vi "ToyForStableDisplayOnGrabberAndSavingData2.vi"() -> ()   [LabVIEW 2010]
panel:
  out "Array of 10":u32[](array[numeric])
  in  "Scanning":bool
  out "appended array":u32[](array[numeric])
  out "Remaining array":u32[](array[numeric])
  in  "stop":bool
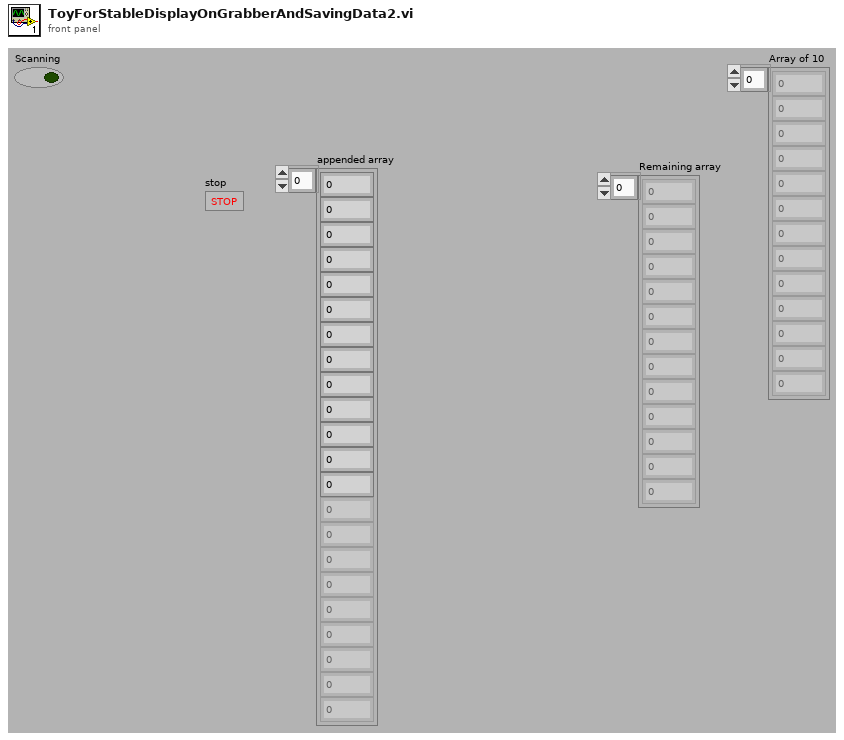
[diagram p1: front panel]
types:
  T1 = enum16{"open", "replace", "create", "open or create", "replace or create", "replace or create with confirmation"}
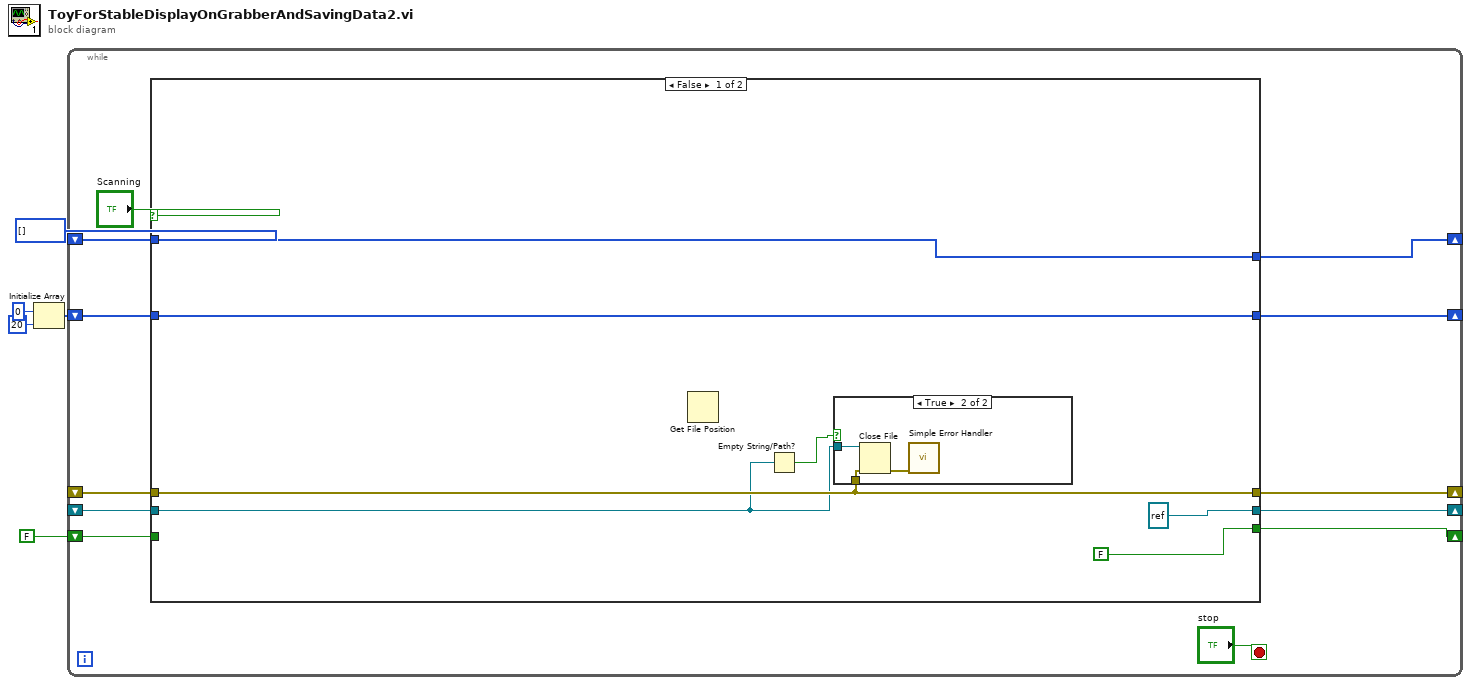
[diagram p0: block diagram]
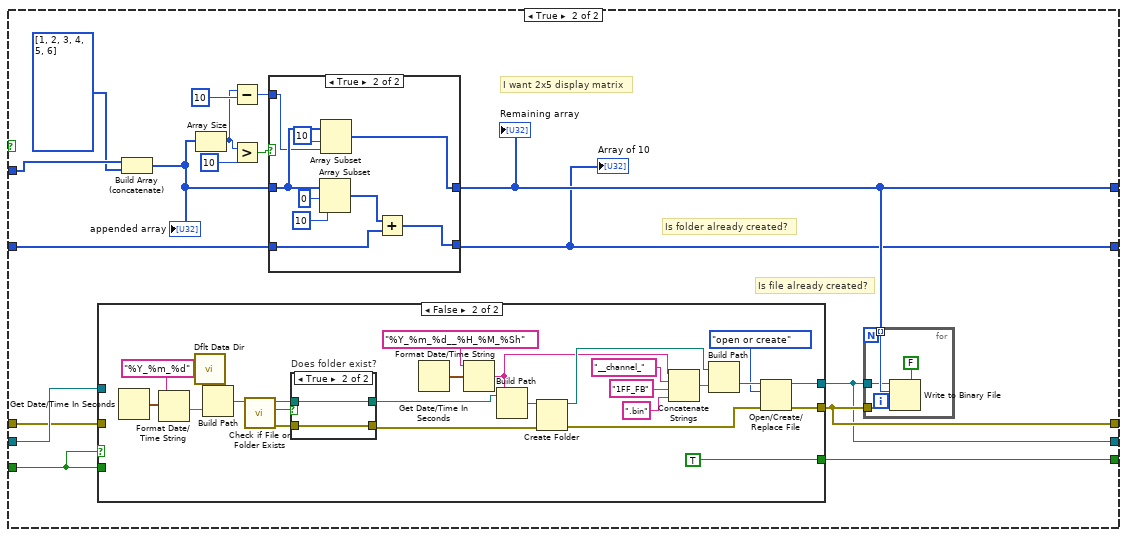
[diagram p3: hidden frame]
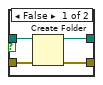
[diagram p5: hidden frame]
diagram:
  n1 = Initialize Array(u32 0 ("element"), 20 ("dimension size")) -> (w2:u32[])
  n2 = while {
    shift-right: [w15] -> _
    shift-left: u32[] [] -> [w16]
    shift-right: [w14] -> _
    shift-left: w2 -> [w13]
    shift-right: [w10] -> _
    shift-left: FALSE -> [w11]
    shift-right: [w9] -> _
    shift-left: _ -> [w8]
    shift-right: [w6] -> _
    shift-left: _ -> [w7]
    stop <- "stop" stop-if-true
    n3 = case shown="False" "Scanning" {
      tunnel: w16 -> [w24 w44]
      tunnel: [w24 w36] -> w15
      tunnel: [w23 w30] -> w14
      tunnel: w13 -> [w23 w37]
      tunnel: w11 -> [_ w34]
      tunnel: [FALSE ("FIFO overflow") w35] -> w10
      tunnel: [refnum<file> refnum ("refnum out") w28] -> w9
      tunnel: w8 -> [w19 w33]
      tunnel: [w21 w29] -> w6
      tunnel: w7 -> [w21 w32]
      frame False {
        n4 = Get File Position() -> ()  [unwired: 2 in, 3 out]
        n5 = Empty String/Path?(string/path=w19) -> (empty?=w18:bool)
        n6 = case shown="True" w18 {
          tunnel: w19 -> [_ w27]
          tunnel: w21 -> [_ w26]
          frame False {
          }
          frame True {
            n7 = Close File(refnum=w27, error in=w26) -> (error out=w25:errorcluster)  [unwired: 1 out]
            n8 = call <vilib>:"Simple Error Handler.vi"("error in (no error)"=w25) -> ()  [unwired: 4 in, 5 out]
          }
        }
      }
      frame True {
        # "Is folder already created?"
        # "Is file already created?"
        # "I want 2x5 display matrix"
        n9 = case shown="False" w34 {
          tunnel: [w50 w52] -> w29
          tunnel: w34 -> [w51 _]
          tunnel: [w51 TRUE ("FIFO overflow")] -> w35
          tunnel: w33 -> [w49 _]
          tunnel: w32 -> [w50 _]
          tunnel: [w49 w54] -> w28
          frame True {
          }
          frame False {
            n10 = Get Date/Time In Seconds() -> (seconds since 1Jan1904=w66:timestamp)
            n11 = Format Date/Time String(time format string (%c)="%Y_%m_%d", seconds (now)=w66) -> (date/time string=w67:string)  [unwired: 1 out]
            n12 = call <vilib>:"Dflt Data Dir.vi"() -> ("App:Default Data Directory"=w61:path)
            n13 = Build Path(base path=w61, name or relative path=w67) -> (appended path=w60:path)
            n14 = call <vilib>:"Check if File or Folder Exists.vi"("path"=w60) -> ("error out"=w62:errorcluster, "file or folder exists?"=w63:bool, "dup path"=w64:path)  [unwired: 1 in, 7 out]
            n15 = case "Does folder exist?" shown="True" w63 {
              tunnel: w62 -> [w80 w82]
              tunnel: w64 -> [w78 w81]
              tunnel: [w79 w82] -> w58
              tunnel: [w77 w81] -> w59
              frame False {
                n16 = Create Folder(path (use dialog)=w78, error in=w80) -> (created path=w77:path, error out=w79:errorcluster)  [unwired: 2 out]
              }
              frame True {
              }
            }
            n17 = Get Date/Time In Seconds() -> (seconds since 1Jan1904=w71:timestamp)
            n18 = Format Date/Time String(time format string (%c)="%Y_%m_%d__%H_%M_%Sh", seconds (now)=w71) -> (date/time string=w68:string)  [unwired: 1 out]
            n19 = Build Path(base path=w59, name or relative path=w68) -> (appended path=w70:path)
            n20 = Create Folder(path (use dialog)=w70, error in=w58) -> (created path=w69:path, error out=w53:errorcluster)  [unwired: 1 in, 1 out]
            n21 = Concatenate Strings(w68, "__channel_" ("string"), "1FF_FB" ("string"), ".bin" ("string")) -> (w73:string)
            n22 = Build Path(base path=w69, name or relative path=w73) -> (appended path=w56:path)
            n23 = Open/Create/Replace File(file path (use dialog)=w56, error in=w53, operation (0:open)=T1."open or create") -> (refnum out=w54:refnum<file>, error out=w52:errorcluster)  [unwired: 3 in, 1 out]
          }
        }
        n24 = Build Array (concatenate)(w44, i32[] [1, 2, 3, 4, 5, 6]) -> (w43:u32[])
        "appended array" <- w43
        n25 = Array Size(array=w43) -> (size(s)=w39:i32)
        n26 = Subtract(x=w39, y=u8 10) -> (x-y=w38:i32)
        n27 = Greater?(x=w39, y=10) -> (0:w41:bool)
        n28 = case shown="True" w41 {
          tunnel: w43 -> [w84 w92]
          tunnel: [w84 w89] -> w36
          tunnel: w38 -> [_ w90]
          tunnel: [w83 w87] -> w30
          tunnel: w37 -> [w83 w85]
          frame False {
          }
          frame True {
            n29 = Array Subset(array=w92, index=0, length=10) -> (w86:u32[])
            n30 = Array Subset(array=w92, index=10, length=w90) -> (w89:u32[])
            n31 = Add(x=w86, y=w85) -> (x+y=w87:u32[])
          }
        }
        "Remaining array" <- w36
        "Array of 10" <- w30
        n32 = for {
          tunnel: w36 -> [w47] mode=indexing
          tunnel: w29 -> [w46]
          tunnel: w28 -> [w45]
          n33 = Write to Binary File(file (use dialog)=w45, data=w47, error in=w46, 5:FALSE ("prepend array or string size? (T)")) -> ()  [unwired: 2 in, 3 out]
        }
      }
    }
  }
